vi "Charger_Check Retry Count and Display Message.vi"(8 "error in":errorcluster, 10 "Charger Inputs":T2 {"setpoint" min=0.0 max=20000.0 step=100.0; "position" min=0 max=5 step=1}, 11 "Status Refnum":T1) -> (0 "error out":errorcluster {"code" format="%.0x"})   [LabVIEW 2020]
uses:
  Drivers/Charger Test Set/Charger_Input Control.ctl
  Charger_Status Refnum.ctl
  Drivers/Charging/Charging_MICS Retry Count.vi
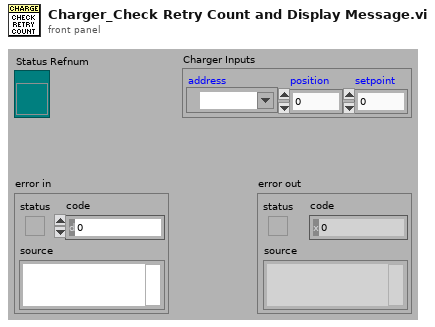
[diagram p1: front panel]
types:
  T1 = typedef "Charger_Status Refnum.ctl" = refnum<vi>
  T2 = typedef "Charger_Input Control.ctl" = cluster{"address":refnum<visa-resource-name>, "position":i32, "setpoint":dbl}
  T3 = cluster{"MICS ID":u32, "VBAT":dbl, "ChargingState":string, "VBAT Slide":dbl, "Status":string, "TemperatureLevel":dbl, "IPG_ReceivedLevel":dbl, "VBAT Target":dbl, "Charger Setpoint":dbl, "Index":i32, "Ready":bool, "Charger Inputs":T2, "MICS Inputs":cluster{"address":refnum<visa-resource-name>, "chan":u16, "ID":u32}}
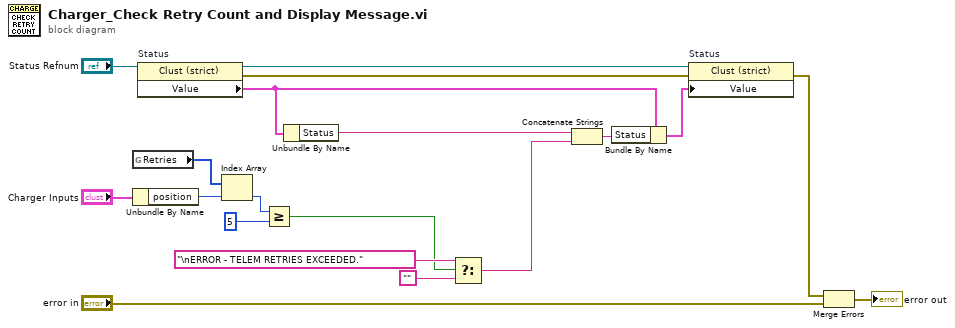
[diagram p0: block diagram]
diagram:
  n1 = global read "Charging_MICS Retry Count.vi" "Retries"() -> (w16:u8[])
  n2 = Unbundle By Name("Charger Inputs") -> ("position"=w17:i32)
  n3 = property on="Status" class="Clust (strict)"(reference="Status Refnum") -> (reference out=w12:T1, error out=w13:errorcluster, "Value"=w11:T3)  [unwired: 1 in]
  n4 = Index Array(array=w16, index=w17) -> (element=w18:u8)
  n5 = Greater Or Equal?(x=w18, y=u8 5) -> (x >= y?=w5:bool)
  n6 = Unbundle By Name(w11) -> ("Status"=w8:string)
  n7 = Select(t="\nERROR - TELEM RETRIES EXCEEDED." ("status message"), s=w5, f="") -> (s? t:f=w4:string)
  n8 = Concatenate Strings(w8, w4) -> (w9:string)
  n9 = Bundle By Name(cluster=w11, "Status"=w9) -> (w10:T3)
  n10 = property on="Status" class="Clust (strict)"(reference=w12, error in=w13, "Value"=w10) -> (error out=w1:errorcluster)  [unwired: 1 out]
  n11 = Merge Errors(w1, "error in") -> (→"error out":errorcluster)
